vi "Test.vi"   [LabVIEW 2018, in "TwinCAT ADS.lvclass"]
uses:
  TwinCAT ADS.lvclass
  TwinCAT.Ads
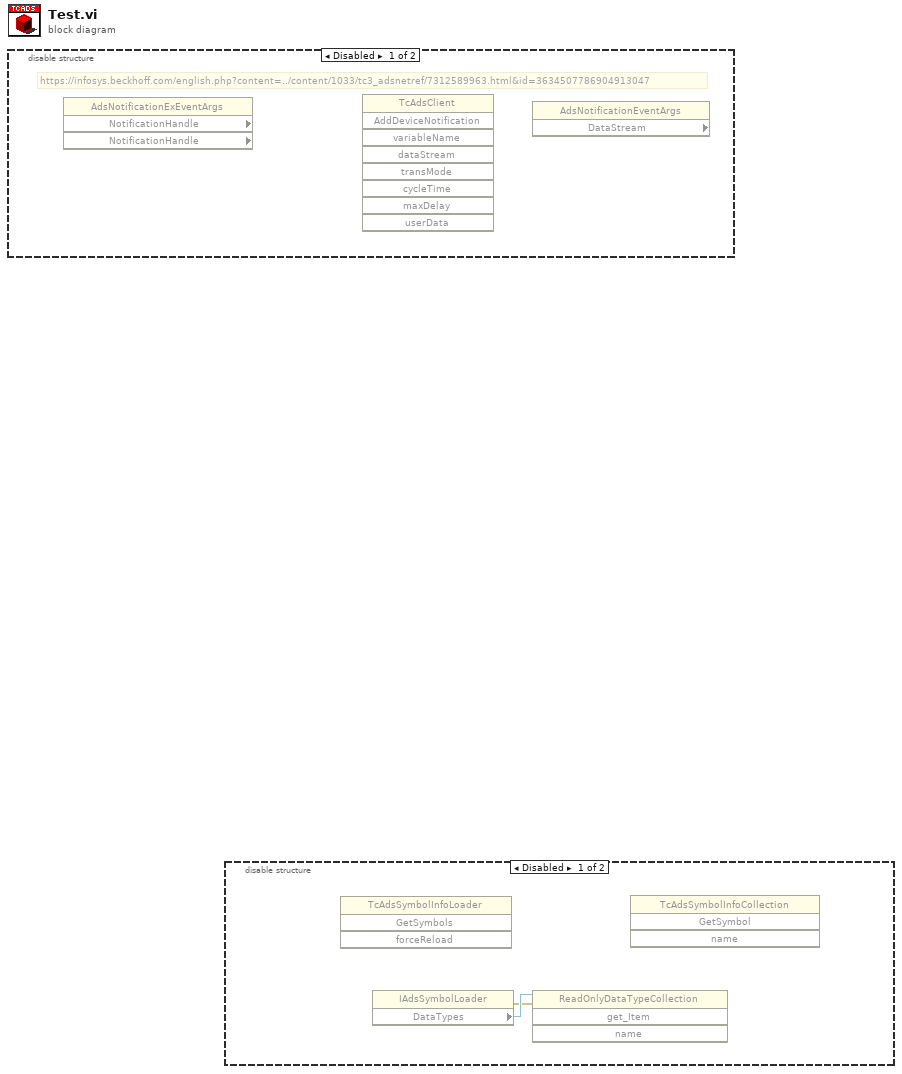
[diagram p0: block diagram]
diagram:
  n1 = disable-structure shown="Disabled" {
    frame Disabled {
      # "https://infosys.beckhoff.com/english.php?content=../content/1033/tc3_adsnetref/7312589963.html&id=3634507786904913047"
      n2 = property class="AdsNotificationExEventArgs" props=["NotificationHandle", "NotificationHandle"]() -> ()  [unwired: 2 in, 4 out]
      n3 = invoke class="TcAdsClient" method="AddDeviceNotification"() -> ()  [unwired: 9 in, 9 out]
      n4 = property class="AdsNotificationEventArgs" props=["DataStream"]() -> ()  [unwired: 2 in, 3 out]
    }
    frame Enabled {
    }
  }
  n5 = disable-structure shown="Disabled" {
    frame Disabled {
      n6 = invoke class="TcAdsSymbolInfoLoader" method="GetSymbols"() -> ()  [unwired: 4 in, 4 out]
      n7 = property class="IAdsSymbolLoader"() -> (error out=w1:errorcluster, "DataTypes"=w2:refnum<k24>)  [unwired: 2 in, 1 out]
      n8 = invoke class="ReadOnlyDataTypeCollection" method="get_Item"(reference=w2, error in=w1) -> ()  [unwired: 2 in, 4 out]
      n9 = invoke class="TcAdsSymbolInfoCollection" method="GetSymbol"() -> ()  [unwired: 4 in, 4 out]
    }
    frame Enabled {
    }
  }
